vi "CRYSet Statistics Front Panel.vi"(11 "Vi Ref":refnum<vi>) -> ()   [LabVIEW 2013]
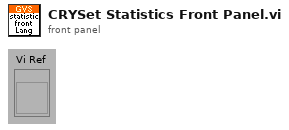
[diagram p1: front panel]
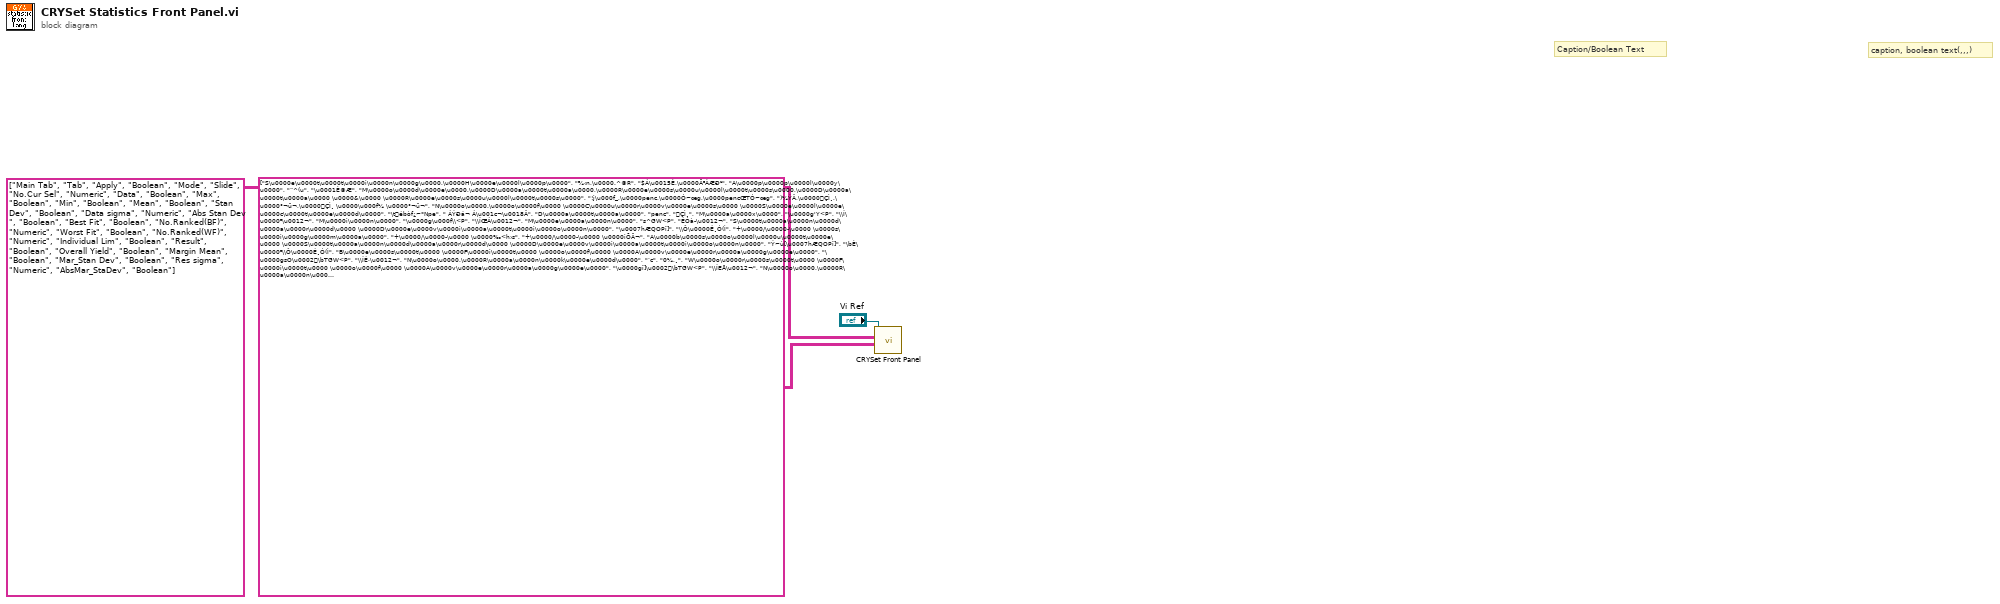
[diagram p0: block diagram]
diagram:
  # "Caption, Tab Page, Multilist Header, Button 4"
  # "Control Type"
  # "Control Name and Tab"
  # "caption, boolean text(,,,)"
  # "Caption/Boolean Text"
  n1 = call "CRYSet Front Panel.vi"("Caption(Boolean Text)"=string[][] [["S\u0000e\u0000t\u0000t\u0000i\u0000n\u0000g\u0000,\u0000H\u0000e\u0000l\u0000p\u0000", "¾‹n,\u0000.^©R", "$Á\u0015È,\u0000Ä³ÀÆÐ¹"], ["A\u0000p\u0000p\u0000l\u0000y\u0000", "”^(u", "\u0001È©Æ"], ["M\u0000o\u0000d\u0000e\u0000,\u0000D\u0000a\u0000t\u0000a\u0000,\u0000R\u0000e\u0000s\u0000u\u0000l\u0000t\u0000s\u0000,\u0000D\u0000a\u0000t\u0000a\u0000 \u0000&\u0000 \u0000R\u0000e\u0000s\u0000u\u0000l\u0000t\u0000s\u0000", "!j\u000f_,\u0000penc,\u0000Ó~œg,\u0000pencŒTÓ~œg", ")¼ÝÂ,\u0000ÇÌ¸,\u0000°¬ü¬,\u0000ÇÌ¸ \u0000\u000f¼ \u0000°¬ü¬"], ["N\u0000o\u0000.\u0000o\u0000f\u0000 \u0000C\u0000u\u0000r\u0000v\u0000e\u0000s\u0000 \u0000S\u0000e\u0000l\u0000e\u0000c\u0000t\u0000e\u0000d\u0000", "\tébòf¿~*Npe", " ÁÝÐá¬ Á\u001c¬\u0018Â"], ["D\u0000a\u0000t\u0000a\u0000", "penc", "ÇÌ¸"], ["M\u0000a\u0000x\u0000", "\u0000g'Y<P", "\\Í\u0000³\u0012¬"], ["M\u0000i\u0000n\u0000", "\u0000g\u000f\\<P", "\\ÍŒÁ\u0012¬"], ["M\u0000e\u0000a\u0000n\u0000", "s^GW<P", "ÉÓà­\u0012¬"], ["S\u0000t\u0000a\u0000n\u0000d\u0000a\u0000r\u0000d\u0000 \u0000D\u0000e\u0000v\u0000i\u0000a\u0000t\u0000i\u0000o\u0000n\u0000", "\u0007hÆQOPî]", "\\Ô\u0000É¸Ó(Ì"], ["+\u0000/\u0000-\u0000 \u0000s\u0000i\u0000g\u0000m\u0000a\u0000", "+\u0000/\u0000-\u0000 \u0000‰<h›s", "+\u0000/\u0000-\u0000 \u0000iÕÄ¬"], ["A\u0000b\u0000s\u0000o\u0000l\u0000u\u0000t\u0000e\u0000 \u0000S\u0000t\u0000a\u0000n\u0000d\u0000a\u0000r\u0000d\u0000 \u0000D\u0000e\u0000v\u0000i\u0000a\u0000t\u0000i\u0000o\u0000n\u0000", "Ý~ù[\u0007hÆQOPî]", "\bÈ\u0000³\\Ô\u0000É¸Ó(Ì"], ["B\u0000e\u0000s\u0000t\u0000 \u0000F\u0000i\u0000t\u0000 \u0000o\u0000f\u0000 \u0000A\u0000v\u0000e\u0000r\u0000a\u0000g\u0000e\u0000", "\u0000gsO\u0002\bTGW<P", "\\ÍÉ·\u0012¬"], ["N\u0000o\u0000.\u0000R\u0000a\u0000n\u0000k\u0000e\u0000d\u0000", "’c", "0¼,¸"], ["W\u0000o\u0000r\u0000s\u0000t\u0000 \u0000F\u0000i\u0000t\u0000 \u0000o\u0000f\u0000 \u0000A\u0000v\u0000e\u0000r\u0000a\u0000g\u0000e\u0000", "\u0000gî]\u0002\bTGW<P", "\\ÍEÅ\u0012¬"], ["N\u0000o\u0000.\u0000R\u0000a\u0000n\u0000k\u0000e\u0000d\u0000", "’c", "ñ´\t®"], ["I\u0000n\u0000d\u0000i\u0000v\u0000i\u0000d\u0000u\u0000a\u0000l\u0000 \u0000L\u0000i\u0000m\u0000i\u0000t\u0000s\u0000 \u0000Y\u0000i\u0000e\u0000l\u0000d\u0000(\u0000%\u0000)\u0000", "USÓ~œg\bT<h(\u0000%\u0000)\u0000", "\u001c¬Ä¼µÑü¬`¹(\u0000%\u0000)\u0000"], ["R\u0000e\u0000s\u0000u\u0000l\u0000t\u0000", "Ó~œg", "°¬ü¬"], ["O\u0000v\u0000e\u0000r\u0000a\u0000l\u0000l\u0000 \u0000Y\u0000i\u0000e\u0000l\u0000d\u0000(\u0000%\u0000)\u0000", ";`\bT<h(\u0000%\u0000)\u0000", "\u0004È´ÌµÑü¬`¹(\u0000%\u0000)\u0000"], ["M\u0000a\u0000r\u0000g\u0000i\u0000n\u0000 \u0000M\u0000e\u0000a\u0000n\u0000", "¹[P–s^GW<P", "½¬Ä¬ÉÓà­\u0012¬"], ["M\u0000a\u0000r\u0000g\u0000i\u0000n\u0000 \u0000S\u0000t\u0000a\u0000n\u0000d\u0000a\u0000r\u0000d\u0000 \u0000D\u0000e\u0000v\u0000i\u0000a\u0000t\u0000i\u0000o\u0000n\u0000", "¹[P–\u0007hÆQî]", "½¬Ä¬\\Ô\u0000É¸Ó(Ì"], ["+\u0000/\u0000-\u0000 \u0000s\u0000i\u0000g\u0000m\u0000a\u0000", "+\u0000/\u0000-\u0000 \u0000‰<h›s", "+\u0000/\u0000-\u0000 \u0000iÕÄ¬"], ["A\u0000b\u0000s\u0000o\u0000l\u0000u\u0000t\u0000e\u0000 \u0000M\u0000a\u0000r\u0000g\u0000i\u0000n\u0000 \u0000S\u0000t\u0000a\u0000n\u0000d\u0000a\u0000r\u0000d\u0000 \u0000D\u0000e\u0000v\u0000i\u0000a\u0000t\u0000i\u0000o\u0000n\u0000", "Ý~ù[¹[P–\u0007hÆQî]", "\bÈ\u0000³½¬Ä¬\\Ô\u0000É¸Ó(Ì"]], "Control ID and Type(Label Name, Type)"=string[][] [["Main Tab", "Tab"], ["Apply", "Boolean"], ["Mode", "Slide"], ["No.Cur Sel", "Numeric"], ["Data", "Boolean"], ["Max", "Boolean"], ["Min", "Boolean"], ["Mean", "Boolean"], ["Stan Dev", "Boolean"], ["Data sigma", "Numeric"], ["Abs Stan Dev ", "Boolean"], ["Best Fit", "Boolean"], ["No.Ranked(BF)", "Numeric"], ["Worst Fit", "Boolean"], ["No.Ranked(WF)", "Numeric"], ["Individual Lim", "Boolean"], ["Result", "Boolean"], ["Overall Yield", "Boolean"], ["Margin Mean", "Boolean"], ["Mar_Stan Dev", "Boolean"], ["Res sigma", "Numeric"], ["AbsMar_StaDev", "Boolean"]], "Vi Ref"="Vi Ref") -> ()  [unwired: 9 in]
